vi "get Last Tx Rx Result.vi"(8 "error in (no error)":errorcluster, 10 "protocol_version":i32, 11 "port_num":i32) -> (0 "error out":errorcluster, 3 "function return":i32)   [LabVIEW 2022 SP3, in "dxl.lvlib"]
doc: "WINDECLSPEC int getLastTxRxResult (int port_num, int protocol_version);"
uses:
  dxl.lvlib
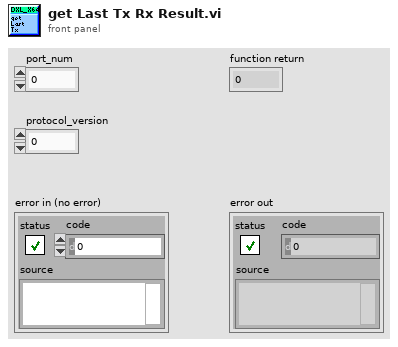
[diagram p1: front panel]
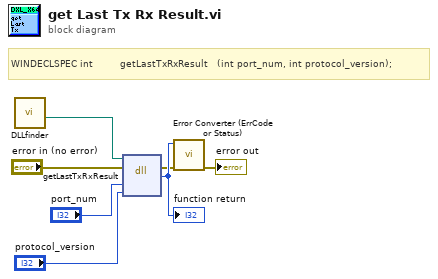
[diagram p0: block diagram]
diagram:
  # "WINDECLSPEC int         getLastTxRxResult   (int port_num, int protocol_version);"
  n1 = call "DLLfinder.vi"() -> ("File Path"=w1:path)  [unwired: 11 in]
  n2 = dll-call lib="C:/EnFlo_Software/ADAM Serial/Instrument drivers/Dynamixel/2nd attempt/Library/dxl_x64_c.*" fn="getLastTxRxResult"(path in=w1, error in="error in (no error)", "port_num"="port_num", "protocol_version"="protocol_version") -> (error out=w3:errorcluster, "return type"=w7:i32)  [unwired: 3 in, 1 out]
  "function return" <- w7
  n3 = call "Error Converter (ErrCode or Status).vi"("error in (no error)"=w3, "error code"=w7) -> ("error out"=→"error out":errorcluster)  [unwired: 9 in]
